vi "Generate_no_B.vi"(8 "error in (no error)":errorcluster, 11 "Button_transfer in":refnum<class "Button_transfer.lvclass">) -> (0 "error out":errorcluster, 3 "Button_transfer out":refnum<class "Button_transfer.lvclass">)   [LabVIEW 2025, in "Button_transfer.lvlib" / "Button_transfer.lvclass"]
uses:
  Button_transfer.lvclass
  Button_transfer.lvclass/Button_transfer.ctl
  B_Actor Messages/Update_random_B Msg/Update_random_B Msg.lvclass/Update_random_B Msg.ctl
  <vilib>/ActorFramework/Message Enqueuer/Message Enqueuer.lvclass/Message Enqueuer.ctl
  <vilib>/numeric/Random Number (Range) U64.vi
  <vilib>/numeric/sub_Random U32.vi
  <vilib>/ActorFramework/Message Enqueuer/Enqueue.vi
  B_Actor Messages/Update_random_B Msg/Update_random_B Msg.lvclass
  C:/Program Files (x86)/National Instruments/LabVIEW 2025/vi.lib/ActorFramework/Message/Message.lvclass
  <vilib>/ActorFramework/Message Priority Queue/Priority Enqueue.vi
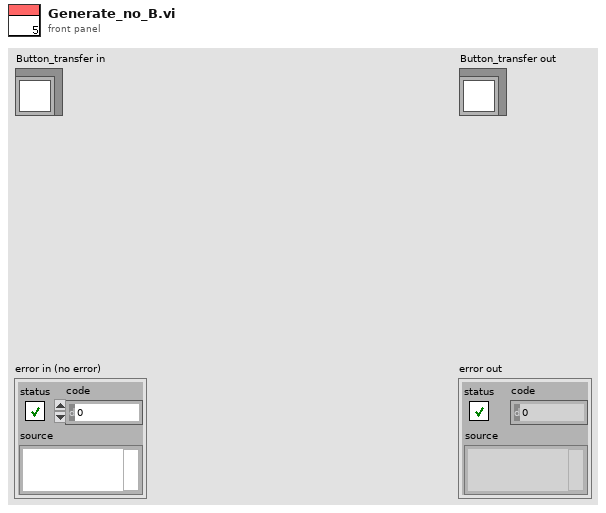
[diagram p1: front panel]
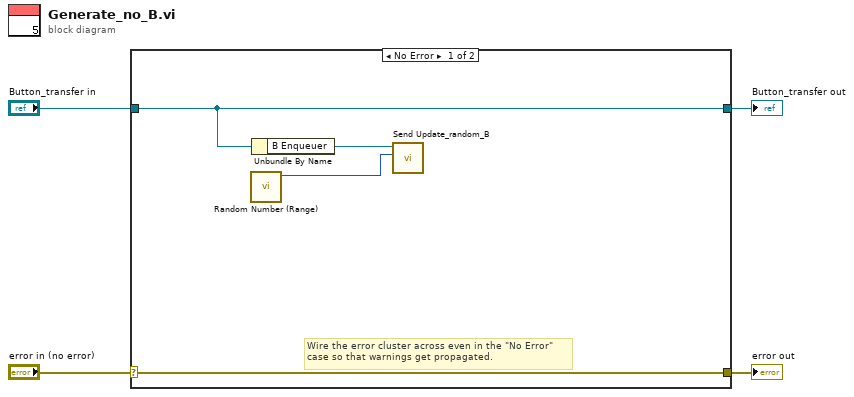
[diagram p0: block diagram]
diagram:
  n1 = case shown="No Error" "error in (no error)" {
    selector: "error in (no error)" -> [w8 w10]
    tunnel: [w8 w10] -> w3
    tunnel: [w7 w9] -> w1
    tunnel: "Button_transfer in" -> [w7 w9]
    frame No Error {
      # "Wire the error cluster across even in the \"No Error\"\ncase so that warnings get propagated."
      n2 = call-poly <vilib>:"Random Number (Range).vi"() -> ("number"=w5:u64)  [unwired: 11 in]
      n3 = Unbundle By Name(w7) -> ("B Enqueuer"=w6:refnum<class "Message Enqueuer.lvclass">)
      n4 = call "Send Update_random_B.vi"("Random"=w5, "Message Enqueuer"=w6) -> ()  [unwired: 8 in, 2 out]
    }
    frame Error {
    }
  }
  "error out" <- w3
  "Button_transfer out" <- w1
